vi "CSTK_Button_Icon_View.vi"(0 "Data In":T21 caption="数据输入", 2 "Display State In":T2={"ButtonSize"={"False"={"Width"=0, "Height"=0}, "True"={"Width"=0, "Height"=0}, "True to False"={"Width"=0, "Height"=0}, "False to True"={"Width"=0, "Height"=0}, "Hover in False"={"Width"=0, "Height"=0}, "Hover in True"={"Width"=0, "Height"=0}}, "Logo Image"={"False"={"image type"=0, "image depth"=0, "image"=[], "mask"=[], "colors"=[], "Rectangle"={"left"=0, "top"=0, "right"=0, "bottom"=0}}, "True"={"image type"=0, "image depth"=0, "image"=[], "mask"=[], "colors"=[], "Rectangle"={"left"=0, "top"=0, "right"=0, "bottom"=0}}, "True to False"={"image type"=0, "image depth"=0, "image"=[], "mask"=[], "colors"=[], "Rectangle"={"left"=0, "top"=0, "right"=0, "bottom"=0}}, "False to True"={"image type"=0, "image depth"=0, "image"=[], "mask"=[], "colors"=[], "Rectangle"={"left"=0, "top"=0, "right"=0, "bottom"=0}}, "Hover in False"={"image type"=0, "image depth"=0, "image"=[], "mask"=[], "colors"=[], "Rectangle"={"left"=0, "top"=0, "right"=0, "bottom"=0}}, "Hover in True"={"image type"=0, "image depth"=0, "image"=[], "mask"=[], "colors"=[], "Rectangle"={"left"=0, "top"=0, "right"=0, "bottom"=0}}}, "Logo Properties"={"False"={"Display Logo?"=FALSE, "Horizontal Offset"=0}, "True"={"Display Logo?"=FALSE, "Horizontal Offset"=0}, "True to False"={"Display Logo?"=FALSE, "Horizontal Offset"=0}, "False to True"={"Display Logo?"=FALSE, "Horizontal Offset"=0}, "Hover in False"={"Display Logo?"=FALSE, "Horizontal Offset"=0}, "Hover in True"={"Display Logo?"=FALSE, "Horizontal Offset"=0}}, "Text String"={"False"="", "True"="", "True to False"="", "False to True"="", "Hover in False"="", "Hover in True"=""}, "Text Properties"={"False"={"Display Text?"=FALSE, "Text Color"=0, "Horizontal Offset"=0, "Font Style"={"Font Name"="", "Size"=0, "Strikeout?"=FALSE, "Italic?"=FALSE, "Underline?"=FALSE, "Outline?"=FALSE, "Shadow?"=FALSE, "Bold?"=FALSE}}, "True"={"Display Text?"=FALSE, "Text Color"=0, "Horizontal Offset"=0, "Font Style"={"Font Name"="", "Size"=0, "Strikeout?"=FALSE, "Italic?"=FALSE, "Underline?"=FALSE, "Outline?"=FALSE, "Shadow?"=FALSE, "Bold?"=FALSE}}, "True to False"={"Display Text?"=FALSE, "Text Color"=0, "Horizontal Offset"=0, "Font Style"={"Font Name"="", "Size"=0, "Strikeout?"=FALSE, "Italic?"=FALSE, "Underline?"=FALSE, "Outline?"=FALSE, "Shadow?"=FALSE, "Bold?"=FALSE}}, "False to True"={"Display Text?"=FALSE, "Text Color"=0, "Horizontal Offset"=0, "Font Style"={"Font Name"="", "Size"=0, "Strikeout?"=FALSE, "Italic?"=FALSE, "Underline?"=FALSE, "Outline?"=FALSE, "Shadow?"=FALSE, "Bold?"=FALSE}}, "Hover in False"={"Display Text?"=FALSE, "Text Color"=0, "Horizontal Offset"=0, "Font Style"={"Font Name"="", "Size"=0, "Strikeout?"=FALSE, "Italic?"=FALSE, "Underline?"=FALSE, "Outline?"=FALSE, "Shadow?"=FALSE, "Bold?"=FALSE}}, "Hover in True"={"Display Text?"=FALSE, "Text Color"=0, "Horizontal Offset"=0, "Font Style"={"Font Name"="", "Size"=0, "Strikeout?"=FALSE, "Italic?"=FALSE, "Underline?"=FALSE, "Outline?"=FALSE, "Shadow?"=FALSE, "Bold?"=FALSE}}}, "BG Color"={"False"=0, "True"=0, "True to False"=0, "False to True"=0, "Hover in False"=0, "Hover in True"=0}, "Border Color"={"False"=0, "True"=0, "True to False"=0, "False to True"=0, "Hover in False"=0, "Hover in True"=0}, "Border Properties"={"False"={"Radius"=0, "Border Style"={"Width"=3, "Style"=enum."Solid"}}, "True"={"Radius"=0, "Border Style"={"Width"=3, "Style"=enum."Solid"}}, "True to False"={"Radius"=0, "Border Style"={"Width"=3, "Style"=enum."Solid"}}, "False to True"={"Radius"=0, "Border Style"={"Width"=3, "Style"=enum."Solid"}}, "Hover in False"={"Radius"=0, "Border Style"={"Width"=3, "Style"=enum."Solid"}}, "Hover in True"={"Radius"=0, "Border Style"={"Width"=3, "Style"=enum."Solid"}}}, "Current BG Image"={"False"=bytes[0], "True"=bytes[0], "True to False"=bytes[0], "False to True"=bytes[0], "Hover in False"=bytes[0], "Hover in True"=bytes[0]}, "DrawAreaSize"={"False"={"Width"=0, "Height"=0}, "True"={"Width"=0, "Height"=0}, "True to False"={"Width"=0, "Height"=0}, "False to True"={"Width"=0, "Height"=0}, "Hover in False"={"Width"=0, "Height"=0}, "Hover in True"={"Width"=0, "Height"=0}}, "Text String Offset"={"False"=0, "True"=0, "True to False"=0, "False to True"=0, "Hover in False"=0, "Hover in True"=0}} caption="显示状态输入", 3 "Container State":T20 caption="容器状态") -> (6 "Data Out":T21 caption="数据输出", 7 "Display State Out":T2={"ButtonSize"={"False"={"Width"=0, "Height"=0}, "True"={"Width"=0, "Height"=0}, "True to False"={"Width"=0, "Height"=0}, "False to True"={"Width"=0, "Height"=0}, "Hover in False"={"Width"=0, "Height"=0}, "Hover in True"={"Width"=0, "Height"=0}}, "Logo Image"={"False"={"image type"=0, "image depth"=0, "image"=[], "mask"=[], "colors"=[], "Rectangle"={"left"=0, "top"=0, "right"=0, "bottom"=0}}, "True"={"image type"=0, "image depth"=0, "image"=[], "mask"=[], "colors"=[], "Rectangle"={"left"=0, "top"=0, "right"=0, "bottom"=0}}, "True to False"={"image type"=0, "image depth"=0, "image"=[], "mask"=[], "colors"=[], "Rectangle"={"left"=0, "top"=0, "right"=0, "bottom"=0}}, "False to True"={"image type"=0, "image depth"=0, "image"=[], "mask"=[], "colors"=[], "Rectangle"={"left"=0, "top"=0, "right"=0, "bottom"=0}}, "Hover in False"={"image type"=0, "image depth"=0, "image"=[], "mask"=[], "colors"=[], "Rectangle"={"left"=0, "top"=0, "right"=0, "bottom"=0}}, "Hover in True"={"image type"=0, "image depth"=0, "image"=[], "mask"=[], "colors"=[], "Rectangle"={"left"=0, "top"=0, "right"=0, "bottom"=0}}}, "Logo Properties"={"False"={"Display Logo?"=FALSE, "Horizontal Offset"=0}, "True"={"Display Logo?"=FALSE, "Horizontal Offset"=0}, "True to False"={"Display Logo?"=FALSE, "Horizontal Offset"=0}, "False to True"={"Display Logo?"=FALSE, "Horizontal Offset"=0}, "Hover in False"={"Display Logo?"=FALSE, "Horizontal Offset"=0}, "Hover in True"={"Display Logo?"=FALSE, "Horizontal Offset"=0}}, "Text String"={"False"="", "True"="", "True to False"="", "False to True"="", "Hover in False"="", "Hover in True"=""}, "Text Properties"={"False"={"Display Text?"=FALSE, "Text Color"=0, "Horizontal Offset"=0, "Font Style"={"Font Name"="", "Size"=0, "Strikeout?"=FALSE, "Italic?"=FALSE, "Underline?"=FALSE, "Outline?"=FALSE, "Shadow?"=FALSE, "Bold?"=FALSE}}, "True"={"Display Text?"=FALSE, "Text Color"=0, "Horizontal Offset"=0, "Font Style"={"Font Name"="", "Size"=0, "Strikeout?"=FALSE, "Italic?"=FALSE, "Underline?"=FALSE, "Outline?"=FALSE, "Shadow?"=FALSE, "Bold?"=FALSE}}, "True to False"={"Display Text?"=FALSE, "Text Color"=0, "Horizontal Offset"=0, "Font Style"={"Font Name"="", "Size"=0, "Strikeout?"=FALSE, "Italic?"=FALSE, "Underline?"=FALSE, "Outline?"=FALSE, "Shadow?"=FALSE, "Bold?"=FALSE}}, "False to True"={"Display Text?"=FALSE, "Text Color"=0, "Horizontal Offset"=0, "Font Style"={"Font Name"="", "Size"=0, "Strikeout?"=FALSE, "Italic?"=FALSE, "Underline?"=FALSE, "Outline?"=FALSE, "Shadow?"=FALSE, "Bold?"=FALSE}}, "Hover in False"={"Display Text?"=FALSE, "Text Color"=0, "Horizontal Offset"=0, "Font Style"={"Font Name"="", "Size"=0, "Strikeout?"=FALSE, "Italic?"=FALSE, "Underline?"=FALSE, "Outline?"=FALSE, "Shadow?"=FALSE, "Bold?"=FALSE}}, "Hover in True"={"Display Text?"=FALSE, "Text Color"=0, "Horizontal Offset"=0, "Font Style"={"Font Name"="", "Size"=0, "Strikeout?"=FALSE, "Italic?"=FALSE, "Underline?"=FALSE, "Outline?"=FALSE, "Shadow?"=FALSE, "Bold?"=FALSE}}}, "BG Color"={"False"=0, "True"=0, "True to False"=0, "False to True"=0, "Hover in False"=0, "Hover in True"=0}, "Border Color"={"False"=0, "True"=0, "True to False"=0, "False to True"=0, "Hover in False"=0, "Hover in True"=0}, "Border Properties"={"False"={"Radius"=0, "Border Style"={"Width"=3, "Style"=enum."Solid"}}, "True"={"Radius"=0, "Border Style"={"Width"=3, "Style"=enum."Solid"}}, "True to False"={"Radius"=0, "Border Style"={"Width"=3, "Style"=enum."Solid"}}, "False to True"={"Radius"=0, "Border Style"={"Width"=3, "Style"=enum."Solid"}}, "Hover in False"={"Radius"=0, "Border Style"={"Width"=3, "Style"=enum."Solid"}}, "Hover in True"={"Radius"=0, "Border Style"={"Width"=3, "Style"=enum."Solid"}}}, "Current BG Image"={"False"=bytes[0], "True"=bytes[0], "True to False"=bytes[0], "False to True"=bytes[0], "Hover in False"=bytes[0], "Hover in True"=bytes[0]}, "DrawAreaSize"={"False"={"Width"=0, "Height"=0}, "True"={"Width"=0, "Height"=0}, "True to False"={"Width"=0, "Height"=0}, "False to True"={"Width"=0, "Height"=0}, "Hover in False"={"Width"=0, "Height"=0}, "Hover in True"={"Width"=0, "Height"=0}}, "Text String Offset"={"False"=0, "True"=0, "True to False"=0, "False to True"=0, "Hover in False"=0, "Hover in True"=0}} caption="显示状态输出", 8 "Action":T1 caption="动作")   [LabVIEW 2015, in "CSTK_Button_Icon.xctl"]
uses:
  CSTK_Button_Icon.xctl
  CSTK_Button_Icon_Data.ctl
  <vilib>/_xctls/Container State.ctl
  CSTK_Button_Icon_Status.ctl
  Private/TypeDefinitions/_CSTK_Button_Icon_ButtonSize.ctl
  <vilib>/Utility/miscctls.llb/LVBoundsTypeDef.ctl
  Private/TypeDefinitions/_CSTK_Button_Icon_LogoImage.ctl
  <vilib>/picture/picture.llb/imagedata.ctl
  Private/TypeDefinitions/_CSTK_Button_Icon_LogoProperties.ctl
  Private/TypeDefinitions/_CSTK_Button_Icon_LogoProperties_Data.ctl
  Private/TypeDefinitions/_CSTK_Button_Icon_TextString.ctl
  Private/TypeDefinitions/_CSTK_Button_Icon_TextProperties.ctl
  Private/TypeDefinitions/_CSTK_Button_Icon_TextProperties_Data.ctl
  Private/TypeDefinitions/_CSTK_Button_Icon_TextProperties_FontStyle.ctl
  Private/TypeDefinitions/_CSTK_Button_Icon_BGColor.ctl
  Private/TypeDefinitions/_CSTK_Button_Icon_BorderColor.ctl
  Private/TypeDefinitions/_CSTK_Button_Icon_BorderProperties.ctl
  Private/TypeDefinitions/_CSTK_Button_Icon_BorderProperties_Data.ctl
  Private/TypeDefinitions/_CSTK_Button_Icon_CurrentBGImage.ctl
  Private/TypeDefinitions/_CSTK_Button_Icon_DrawAreaSize.ctl
  Private/TypeDefinitions/_CSTK_Button_Icon_TextStartOffset.ctl
  <vilib>/_xctls/Action.ctl
  Private/TypeDefinitions/_CSTK_Button_Icon_EventData.ctl
  <vilib>/_xctls/XControlSupport.lvlib
panel:
  out "CSTK_Button":picture
types:
  T1 = typedef "XControlSupport.lvlib/Action.ctl" = cluster{"Data Changed?":bool, "State Changed?":bool, "Action Name":string}
  T2 = typedef "CSTK_Button_Icon.xctl/CSTK_Button_Icon_Status.ctl" = cluster{"ButtonSize":T3, "Logo Image":T5, "Logo Properties":T7, "Text String":T9, "Text Properties":T10, "BG Color":T13, "Border Color":T14, "Border Properties":T15, "Current BG Image":T17, "DrawAreaSize":T18, "Text String Offset":T19}
  T3 = typedef "CSTK_Button_Icon.xctl/_CSTK_Button_Icon_ButtonSize.ctl" = cluster{"False":T4, "True":T4, "True to False":T4, "False to True":T4, "Hover in False":T4, "Hover in True":T4}
  T4 = typedef "LVBoundsTypeDef.ctl" = cluster{"Width":u32, "Height":u32}
  T5 = typedef "CSTK_Button_Icon.xctl/_CSTK_Button_Icon_LogoImage.ctl" = cluster{"False":T6, "True":T6, "True to False":T6, "False to True":T6, "Hover in False":T6, "Hover in True":T6}
  T6 = typedef "imagedata.ctl" = cluster{"image type":i32, "image depth":i32, "image":u8[], "mask":u8[], "colors":u32[], "Rectangle":cluster{"left":i16, "top":i16, "right":i16, "bottom":i16}}
  T7 = typedef "CSTK_Button_Icon.xctl/_CSTK_Button_Icon_LogoProperties.ctl" = cluster{"False":T8, "True":T8, "True to False":T8, "False to True":T8, "Hover in False":T8, "Hover in True":T8}
  T8 = typedef "CSTK_Button_Icon.xctl/_CSTK_Button_Icon_LogoProperties_Data.ctl" = cluster{"Display Logo?":bool, "Horizontal Offset":i16}
  T9 = typedef "CSTK_Button_Icon.xctl/_CSTK_Button_Icon_TextString.ctl" = cluster{"False":string, "True":string, "True to False":string, "False to True":string, "Hover in False":string, "Hover in True":string}
  T10 = typedef "CSTK_Button_Icon.xctl/_CSTK_Button_Icon_TextProperties.ctl" = cluster{"False":T11, "True":T11, "True to False":T11, "False to True":T11, "Hover in False":T11, "Hover in True":T11}
  T11 = typedef "CSTK_Button_Icon.xctl/_CSTK_Button_Icon_TextProperties_Data.ctl" = cluster{"Display Text?":bool, "Text Color":u32, "Horizontal Offset":i16, "Font Style":T12}
  T12 = typedef "CSTK_Button_Icon.xctl/_CSTK_Button_Icon_TextProperties_FontStyle.ctl" = cluster{"Font Name":string, "Size":i16, "Strikeout?":bool, "Italic?":bool, "Underline?":bool, "Outline?":bool, "Shadow?":bool, "Bold?":bool}
  T13 = typedef "CSTK_Button_Icon.xctl/_CSTK_Button_Icon_BGColor.ctl" = cluster{"False":u32, "True":u32, "True to False":u32, "False to True":u32, "Hover in False":u32, "Hover in True":u32}
  T14 = typedef "CSTK_Button_Icon.xctl/_CSTK_Button_Icon_BorderColor.ctl" = cluster{"False":u32, "True":u32, "True to False":u32, "False to True":u32, "Hover in False":u32, "Hover in True":u32}
  T15 = typedef "CSTK_Button_Icon.xctl/_CSTK_Button_Icon_BorderProperties.ctl" = cluster{"False":T16, "True":T16, "True to False":T16, "False to True":T16, "Hover in False":T16, "Hover in True":T16}
  T16 = typedef "CSTK_Button_Icon.xctl/_CSTK_Button_Icon_BorderProperties_Data.ctl" = cluster{"Radius":i16, "Border Style":cluster{"Width":u16, "Style":enum32{"Solid", "Dash", "Dot", "DashDot", "DashDotDot"}}}
  T17 = typedef "CSTK_Button_Icon.xctl/_CSTK_Button_Icon_CurrentBGImage.ctl" = cluster{"False":picture, "True":picture, "True to False":picture, "False to True":picture, "Hover in False":picture, "Hover in True":picture}
  T18 = typedef "CSTK_Button_Icon.xctl/_CSTK_Button_Icon_DrawAreaSize.ctl" = cluster{"False":T4, "True":T4, "True to False":T4, "False to True":T4, "Hover in False":T4, "Hover in True":T4}
  T19 = typedef "CSTK_Button_Icon.xctl/_CSTK_Button_Icon_TextStartOffset.ctl" = cluster{"False":i32, "True":i32, "True to False":i32, "False to True":i32, "Hover in False":i32, "Hover in True":i32}
  T20 = typedef "XControlSupport.lvlib/Container State.ctl" = cluster{"Indicator?":bool, "Run Mode?":bool, " Refnum":refnum<vi>}
  T21 = typedef "CSTK_Button_Icon.xctl/CSTK_Button_Icon_Data.ctl" = bool
  T22 = typedef "CSTK_Button_Icon.xctl/_CSTK_Button_Icon_EventData.ctl" = cluster{"BGImage":picture, "DrawAreaSize":T4, "UpdateDrawArea":bool, "调用方":string}
  T23 = typedef "LVRectTypeDef.ctl" = cluster{"Left":i16, "Top":i16, "Right":i16, "Bottom":i16}
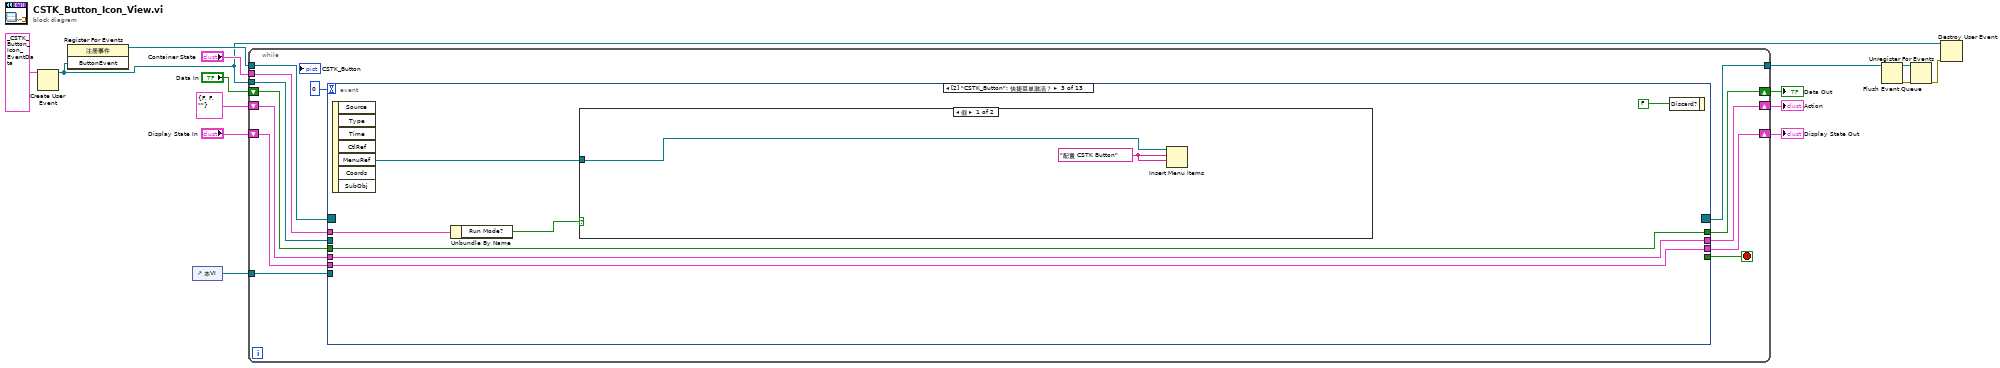
[diagram p0: block diagram]
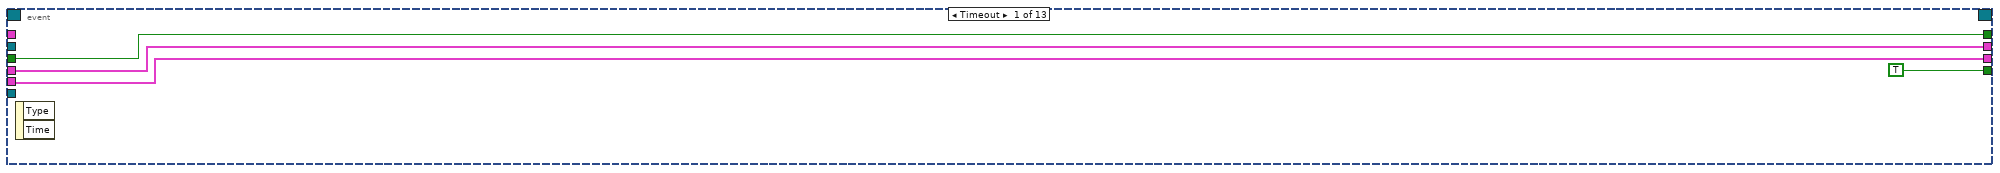
[diagram p2: hidden frame]
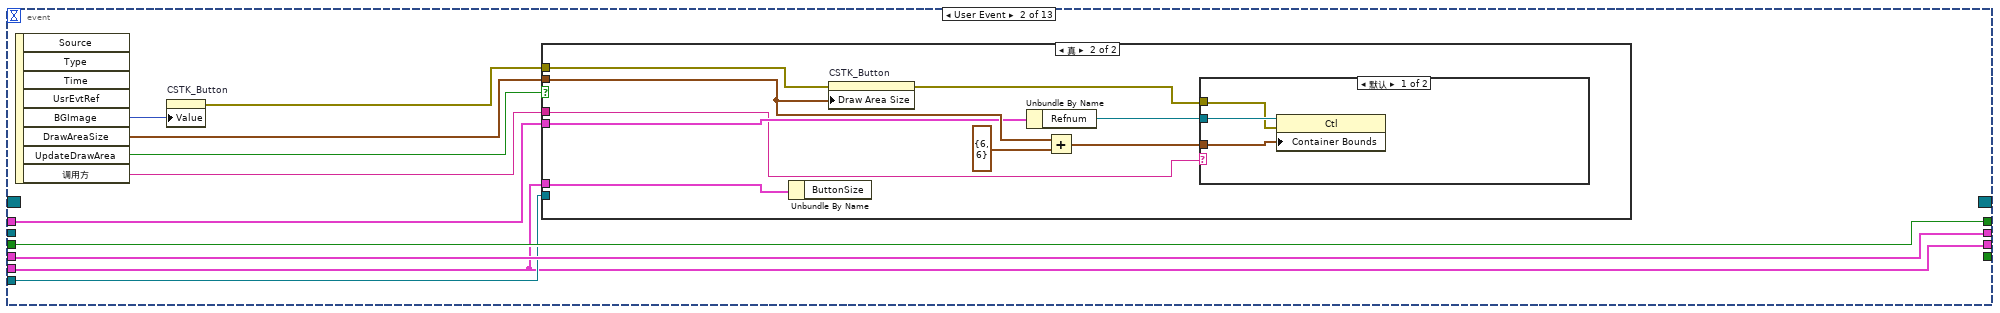
[diagram p3: hidden frame]
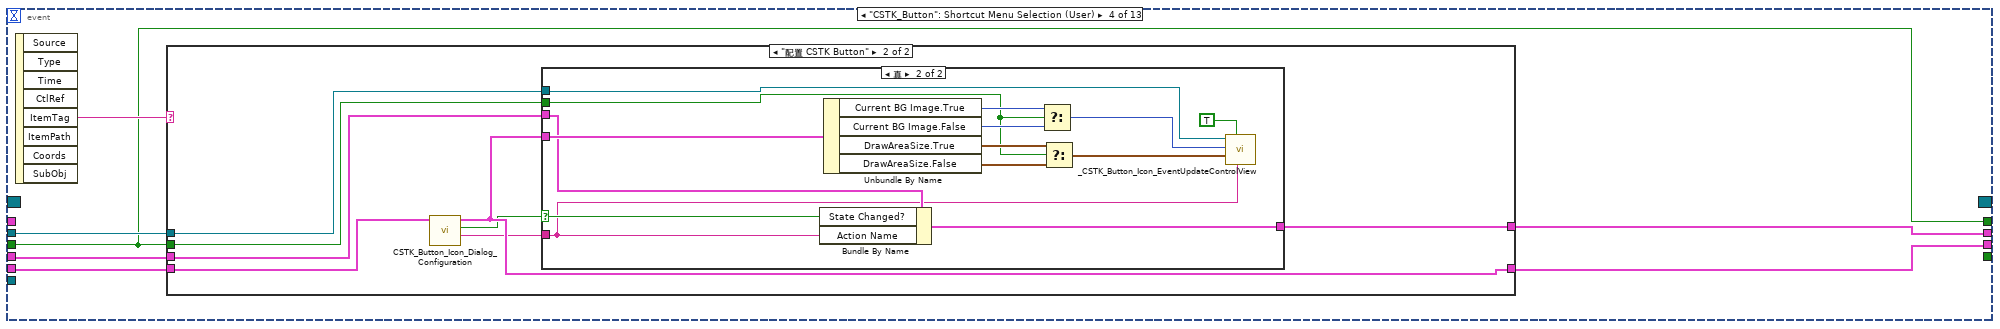
[diagram p7: hidden frame]
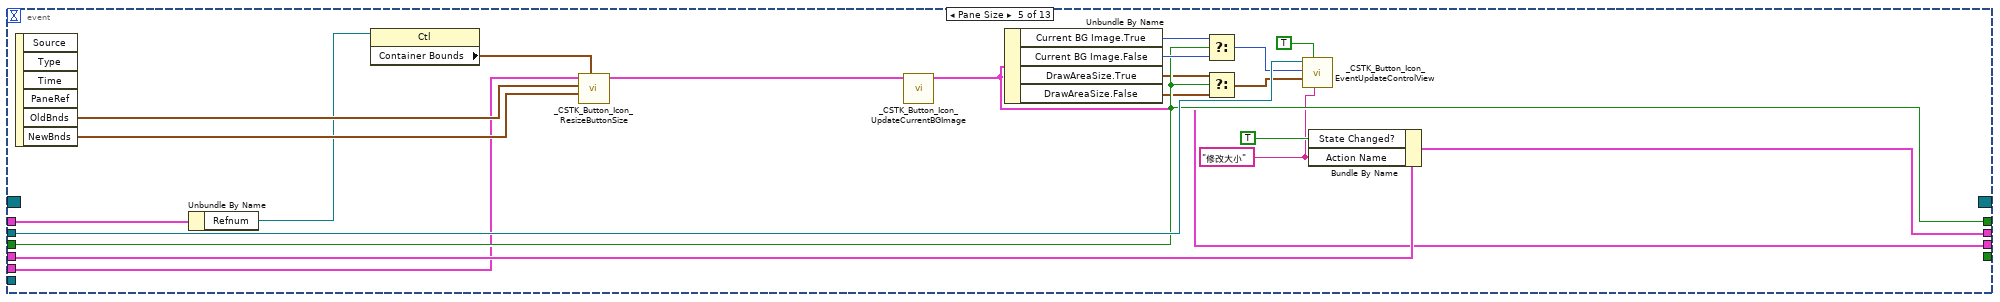
[diagram p10: hidden frame]
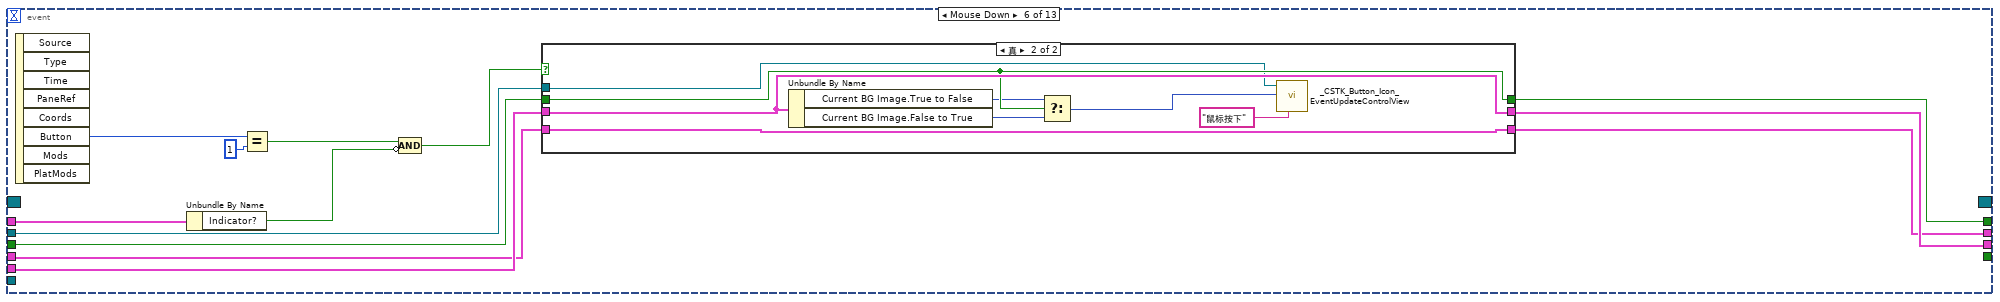
[diagram p11: hidden frame]
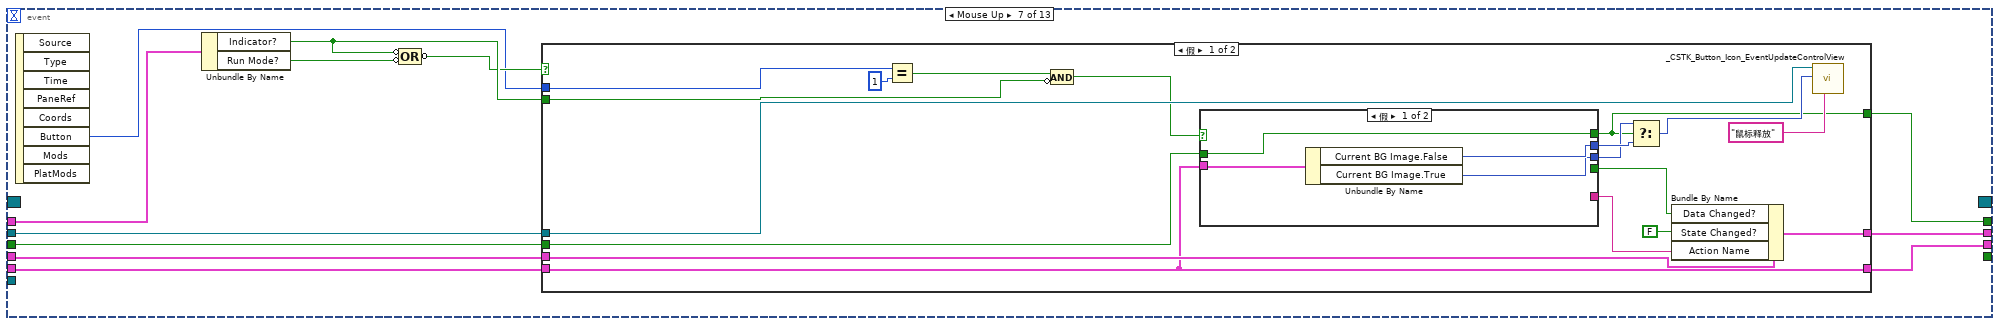
[diagram p13: hidden frame]
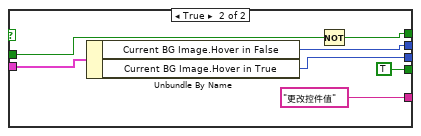
[diagram p14: hidden frame]
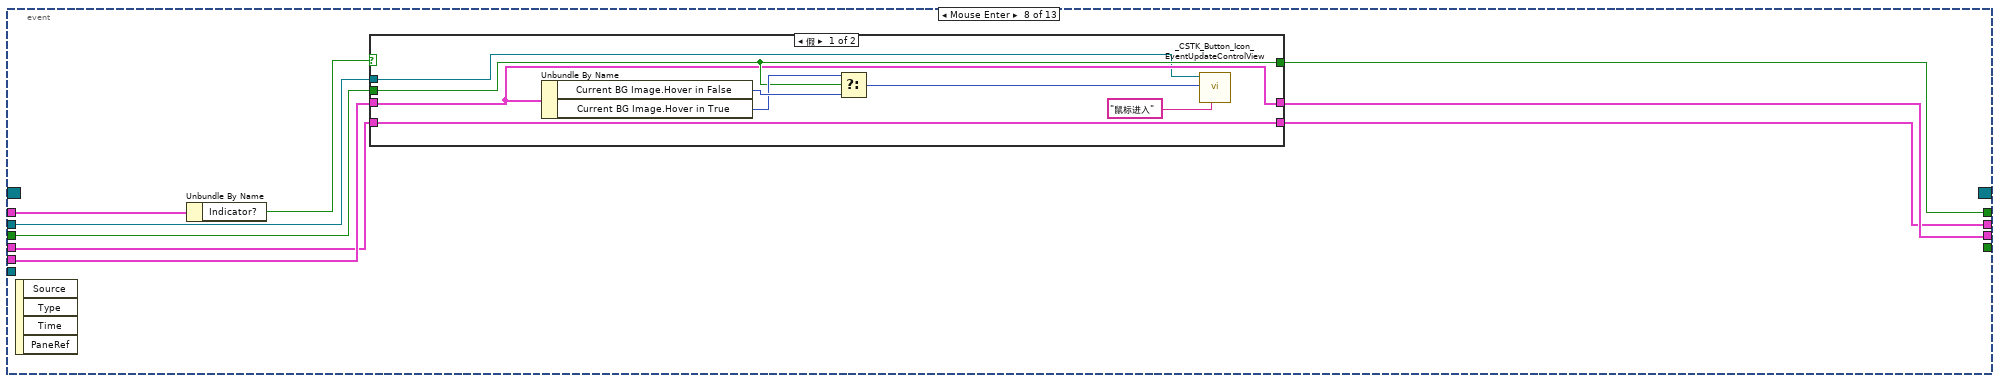
[diagram p16: hidden frame]
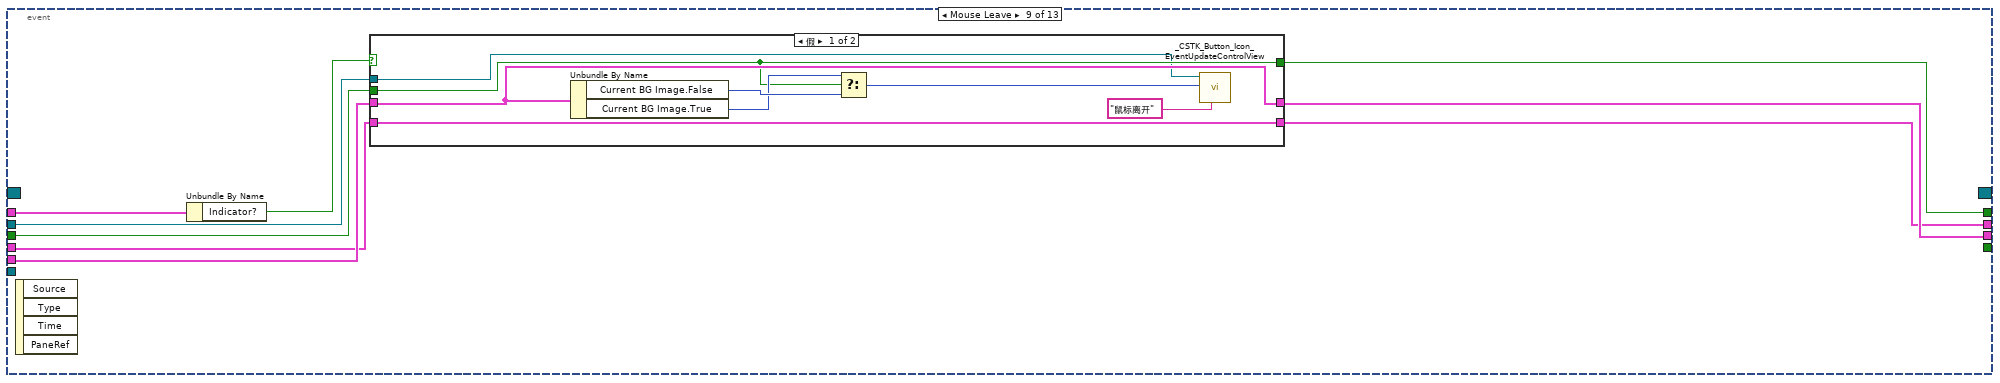
[diagram p18: hidden frame]
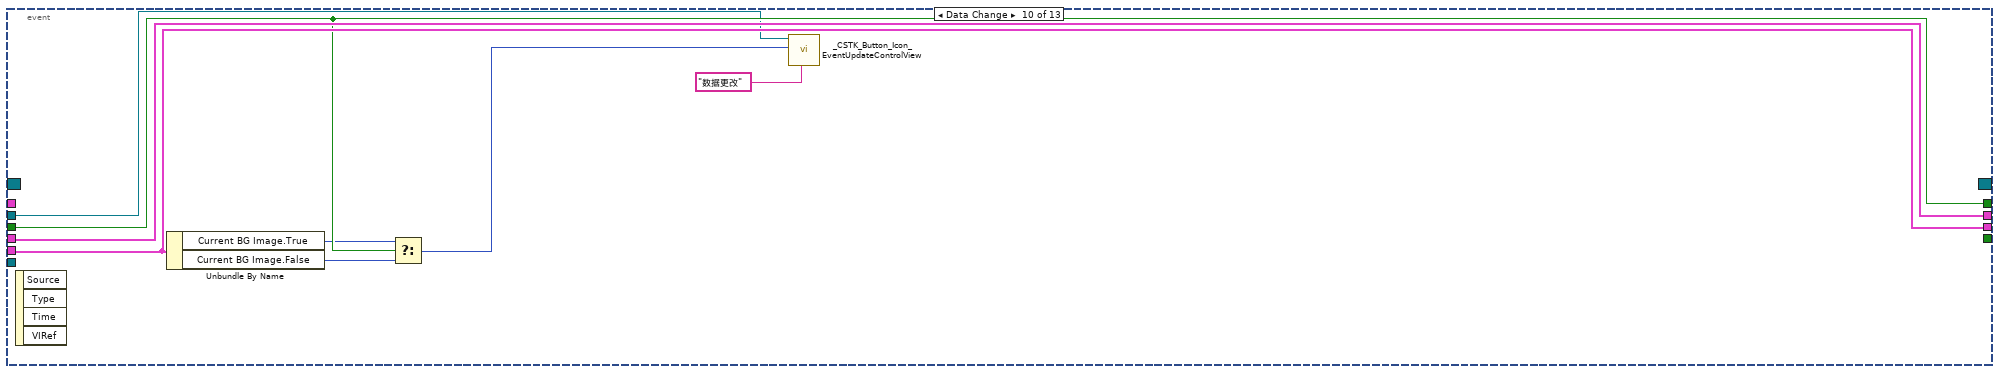
[diagram p20: hidden frame]
diagram:
  n1 = Create User Event(user event datatype=T22 {"BGImage"=bytes[0], "DrawAreaSize"={"Width"=0, "Height"=0}, "UpdateDrawArea"=FALSE, "调用方"=""} ("ButtonEvent")) -> (user event=w2:refnum<user-event>)  [unwired: 1 in, 1 out]
  n2 = register-events(w2) -> (reference out=w6:refnum<event-registration>)  [unwired: 2 in, 1 out]
  n3 = control-ref of="本VI"() -> (w8:refnum<vi>)
  n4 = while {
    shift-right: [w27] -> w12
    shift-left: "Display State In" -> [w28]
    tunnel: "Container State" -> [w24]
    shift-right: [w22] -> w15
    shift-left: "Data In" -> [w23]
    shift-right: [w20] -> w10
    shift-left: T1 {"Data Changed?"=FALSE, "State Changed?"=FALSE, "Action Name"=""} ("Action") -> [w21]
    tunnel: w8 -> [w19]
    tunnel: w6 -> [w18]
    tunnel: w2 -> [w16]
    tunnel: [w17] -> w5
    stop <- w26 stop-if-true
    n5 = event shown="[2] \"CSTK_Button\": 快捷菜单激活？" {
      selector: w18 -> [_ _ _ _ _ _ _ _ _ _ _ _ _]
      dyn-events: [_ _ _ _ _ _ _ _ _ _ _ _ _] -> w17
      timeout: 0 -> [_ _ _ _ _ _ _ _ _ _ _ _ _]
      tunnel: w28 -> [w30 w33 w61 w69 w102 w127 w150 w191 w211 w231 w233 w245 w257]
      tunnel: [w30 w33 w61 w68 w100 w126 w149 w190 w210 w231 w233 w245 w257] -> w27
      tunnel: [TRUE _ _ _ _ _ _ _ _ _ _ _ _] -> w26
      tunnel: w24 -> [_ w35 w56 _ w99 w123 w146 w187 w207 _ _ w251 w258]
      tunnel: w23 -> [w29 w42 w60 w66 w107 w129 w152 w193 w213 w230 w243 w250 w256]
      tunnel: [w29 w42 w60 w66 w107 w128 w151 w192 w212 w230 w243 w250 w256] -> w22
      tunnel: [w31 w41 w59 w64 w115 w124 w147 w188 w208 w232 w244 w248 w254] -> w20
      tunnel: w21 -> [w31 w41 w59 w65 w116 w125 w148 w189 w209 w232 w244 w249 w255]
      tunnel: w19 -> [_ w36 _ _ _ _ _ _ _ _ _ _ _]
      tunnel: w16 -> [_ _ _ w67 w111 w121 w142 w185 w205 w227 w238 _ _]
      event Timeout {
        n6 = event-data() -> ()  [unwired: 1 in, 2 out]
      }
      event User Event {
        n7 = event-data() -> ("BGImage"=w40:picture, "DrawAreaSize"=w38:T4, "UpdateDrawArea"=w37:bool, "调用方"=w34:string)  [unwired: 1 in, 4 out]
        n8 = property on="CSTK_Button" class="Pict"("Value"=w40) -> (error out=w39:errorcluster)  [unwired: 2 in, 1 out]
        n9 = case shown="真" w37 {
          tunnel: w39 -> [_ w51]
          tunnel: w38 -> [_ w49]
          tunnel: w36 -> [_ _]
          tunnel: w35 -> [_ w48]
          tunnel: w34 -> [_ w44]
          tunnel: w33 -> [_ w43]
          frame False {
          }
          frame True {
            n10 = Unbundle By Name(w43) -> ()  [unwired: 1 out]
            n11 = property on="CSTK_Button" class="Pict"(error in=w51, "Draw Area Size"=w49) -> (error out=w46:errorcluster)  [unwired: 1 in, 1 out]
            n12 = Unbundle By Name(w48) -> ("Refnum"=w45:refnum<vi>)
            n13 = Add(x=w49, y=T4 {"Width"=6, "Height"=6}) -> (x+y=w47:T4)
            n14 = case shown="默认" w44 {
              tunnel: w47 -> [w52 _]
              tunnel: w45 -> [w54 _]
              tunnel: w46 -> [w53 _]
              frame Default {
                n15 = property class="Ctl"(reference=w54, error in=w53, "Container Bounds"=w52) -> ()  [unwired: 2 out]
              }
              frame "修改大小" {
              }
            }
          }
        }
      }
      event "CSTK_Button": Shortcut Menu Activation? {
        n16 = event-data() -> ("MenuRef"=w58:refnum<k9>)  [unwired: 1 in, 6 out]
        n17 = Unbundle By Name(w56) -> ("Run Mode?"=w55:bool)
        n18 = case shown="假" w55 {
          tunnel: w58 -> [w62 _]
          frame False {
            w63 = "配置 CSTK Button"
            n19 = Insert Menu Items(7:w63, 8:w63, 9:w62) -> ()  [unwired: 3 in, 3 out]
          }
          frame True {
          }
        }
        n20 = event-data("Discard?"=FALSE ("放弃？")) -> ()  [unwired: 1 in, 1 out]
      }
      event "CSTK_Button": Shortcut Menu Selection (User) {
        n21 = event-data() -> ("ItemTag"=w70:string)  [unwired: 1 in, 7 out]
        n22 = case shown="\"配置 CSTK Button\"" w70 {
          tunnel: w69 -> [w72 w80]
          tunnel: [w72 w78] -> w68
          tunnel: w67 -> [_ w79]
          tunnel: w66 -> [_ w77]
          tunnel: [w71 w73] -> w64
          tunnel: w65 -> [w71 w74]
          frame Default {
          }
          frame "配置 CSTK Button" {
            n23 = call "CSTK_Button_Icon_Dialog_Configuration.vi"("State in"=w80) -> ("Action Name"=w76:string, "State Changed?"=w75:bool, "State out"=w78:T2)  [unwired: 8 in]
            n24 = case shown="真" w75 {
              selector: w75 -> [_ w84]
              tunnel: w79 -> [_ w88]
              tunnel: w78 -> [_ w87]
              tunnel: w76 -> [_ w83]
              tunnel: w77 -> [_ w86]
              tunnel: w74 -> [w81 w85]
              tunnel: [w81 w82] -> w73
              frame False {
              }
              frame True {
                n25 = Bundle By Name(cluster=w85, "State Changed?"=w84, "Action Name"=w83) -> (w82:T1)
                n26 = Unbundle By Name(w87) -> ("Current BG Image.True"=w95:picture, "Current BG Image.False"=w94:picture, "DrawAreaSize.True"=w93:T4, "DrawAreaSize.False"=w92:T4)
                n27 = Select(t=w95, s=w86, f=w94) -> (s? t:f=w91:picture)
                n28 = Select(t=w93, s=w86, f=w92) -> (s? t:f=w90:T4)
                n29 = call "_CSTK_Button_Icon_EventUpdateControlView.vi"("调用方"=w83, "UpdateDrawArea"=TRUE, "DrawAreaSize"=w90, "BGImage"=w91, "用户事件输入"=w88) -> ()  [unwired: 5 in, 2 out]
              }
            }
          }
        }
      }
      event Pane Size {
        w96 = "修改大小" ("Action Name")
        n30 = event-data() -> ("OldBnds"=w113:T23, "NewBnds"=w112:T23)  [unwired: 1 in, 4 out]
        n31 = Unbundle By Name(w99) -> ("Refnum"=w98:refnum<vi>)
        n32 = property class="Ctl"(reference=w98) -> ("Container Bounds"=w97:T4)  [unwired: 1 in, 2 out]
        n33 = call "_CSTK_Button_Icon_ResizeButtonSize.vi"("XControl:容器边界"=w97, "NewBnds"=w112, "OldBnds"=w113, "Display State 输入"=w102) -> ("Display State 输出"=w101:T2)  [unwired: 7 in]
        n34 = call "_CSTK_Button_Icon_UpdateCurrentBGImage.vi"("State in"=w101) -> ("State out"=w100:T2)  [unwired: 10 in]
        n35 = Unbundle By Name(w100) -> ("Current BG Image.True"=w110:picture, "Current BG Image.False"=w109:picture, "DrawAreaSize.True"=w106:T4, "DrawAreaSize.False"=w105:T4)
        n36 = Select(t=w110, s=w107, f=w109) -> (s? t:f=w108:picture)
        n37 = Select(t=w106, s=w107, f=w105) -> (s? t:f=w104:T4)
        n38 = call "_CSTK_Button_Icon_EventUpdateControlView.vi"("调用方"=w96, "UpdateDrawArea"=TRUE, "DrawAreaSize"=w104, "BGImage"=w108, "用户事件输入"=w111) -> ()  [unwired: 5 in, 2 out]
        n39 = Bundle By Name(cluster=w116, "State Changed?"=TRUE, "Action Name"=w96) -> (w115:T1)
      }
      event Mouse Down {
        n40 = event-data() -> ("Button"=w119:u16)  [unwired: 1 in, 7 out]
        n41 = Unbundle By Name(w123) -> ("Indicator?"=w122:bool)
        n42 = Equal?(x=w119, y=u16 1) -> (x = y?=w117:bool)
        n43 = Compound Arithmetic op=AND ("复合运算")(w117, invert w122) -> (w120:bool)
        n44 = case shown="真" w120 {
          tunnel: w129 -> [w132 w139]
          tunnel: [w132 w139] -> w128
          tunnel: w127 -> [w131 w140]
          tunnel: [w131 w140] -> w126
          tunnel: w125 -> [w130 w136]
          tunnel: [w130 w136] -> w124
          tunnel: w121 -> [_ w135]
          frame False {
          }
          frame True {
            n45 = Unbundle By Name(w140) -> ("Current BG Image.True to False"=w138:picture, "Current BG Image.False to True"=w137:picture)
            n46 = Select(t=w138, s=w139, f=w137) -> (s? t:f=w134:picture)
            n47 = call "_CSTK_Button_Icon_EventUpdateControlView.vi"("调用方"="鼠标按下", "BGImage"=w134, "用户事件输入"=w135) -> ()  [unwired: 7 in, 2 out]
          }
        }
      }
      event Mouse Up {
        n48 = event-data() -> ("Button"=w141:u16)  [unwired: 1 in, 7 out]
        n49 = Unbundle By Name(w146) -> ("Indicator?"=w145:bool, "Run Mode?"=w144:bool)
        n50 = Compound Arithmetic op=OR ("复合运算")(invert w145, invert w144) -> (invert w143:bool)
        n51 = case shown="假" w143 {
          tunnel: w152 -> [w156 w184]
          tunnel: [w155 w184] -> w151
          tunnel: w150 -> [w167 w183]
          tunnel: [w167 w183] -> w149
          tunnel: w148 -> [w170 w182]
          tunnel: [w169 w182] -> w147
          tunnel: w145 -> [w164 _]
          tunnel: w142 -> [w163 _]
          tunnel: w141 -> [w159 _]
          frame False {
            n52 = Equal?(x=w159, y=u16 1) -> (x = y?=w157:bool)
            n53 = Compound Arithmetic op=AND ("复合运算")(w157, invert w164) -> (w160:bool)
            n54 = case shown="假" w160 {
              tunnel: w167 -> [w174 w181]
              tunnel: [w173 w180] -> w166
              tunnel: [w172 w179] -> w165
              tunnel: w156 -> [w171 w178]
              tunnel: [w171 w177] -> w155
              tunnel: [_ TRUE ("Data Changed?")] -> w154
              tunnel: [_ "更改控件值" ("Action Name")] -> w153
              frame False {
                n55 = Unbundle By Name(w174) -> ("Current BG Image.False"=w173:picture, "Current BG Image.True"=w172:picture)
              }
              frame True {
                n56 = Unbundle By Name(w181) -> ("Current BG Image.Hover in False"=w180:picture, "Current BG Image.Hover in True"=w179:picture)
                n57 = Not(x=w178) -> (.not. x?=w177:T21)
              }
            }
            n58 = Select(t=w165, s=w155, f=w166) -> (s? t:f=w162:picture)
            n59 = Bundle By Name(cluster=w170, "Data Changed?"=w154, "State Changed?"=FALSE, "Action Name"=w153) -> (w169:T1)
            n60 = call "_CSTK_Button_Icon_EventUpdateControlView.vi"("调用方"="鼠标释放", "BGImage"=w162, "用户事件输入"=w163) -> ()  [unwired: 7 in, 2 out]
          }
          frame True {
          }
        }
      }
      event Mouse Enter {
        n61 = event-data() -> ()  [unwired: 1 in, 4 out]
        n62 = Unbundle By Name(w187) -> ("Indicator?"=w186:bool)
        n63 = case shown="假" w186 {
          tunnel: w193 -> [w198 w204]
          tunnel: [w198 w204] -> w192
          tunnel: w191 -> [w197 w203]
          tunnel: [w197 w203] -> w190
          tunnel: w189 -> [w201 w202]
          tunnel: [w201 w202] -> w188
          tunnel: w185 -> [w195 _]
          frame False {
            n64 = Unbundle By Name(w197) -> ("Current BG Image.Hover in False"=w200:picture, "Current BG Image.Hover in True"=w199:picture)
            n65 = Select(t=w199, s=w198, f=w200) -> (s? t:f=w196:picture)
            n66 = call "_CSTK_Button_Icon_EventUpdateControlView.vi"("调用方"="鼠标进入", "BGImage"=w196, "用户事件输入"=w195) -> ()  [unwired: 7 in, 2 out]
          }
          frame True {
          }
        }
      }
      event Mouse Leave {
        n67 = event-data() -> ()  [unwired: 1 in, 4 out]
        n68 = Unbundle By Name(w207) -> ("Indicator?"=w206:bool)
        n69 = case shown="假" w206 {
          tunnel: w213 -> [w217 w224]
          tunnel: [w217 w224] -> w212
          tunnel: w211 -> [w220 w223]
          tunnel: [w220 w223] -> w210
          tunnel: w209 -> [w221 w222]
          tunnel: [w221 w222] -> w208
          tunnel: w205 -> [w215 _]
          frame False {
            n70 = Unbundle By Name(w220) -> ("Current BG Image.False"=w219:picture, "Current BG Image.True"=w218:picture)
            n71 = Select(t=w218, s=w217, f=w219) -> (s? t:f=w216:picture)
            n72 = call "_CSTK_Button_Icon_EventUpdateControlView.vi"("调用方"="鼠标离开", "BGImage"=w216, "用户事件输入"=w215) -> ()  [unwired: 7 in, 2 out]
          }
          frame True {
          }
        }
      }
      event Data Change {
        n73 = event-data() -> ()  [unwired: 1 in, 4 out]
        n74 = Unbundle By Name(w231) -> ("Current BG Image.True"=w229:picture, "Current BG Image.False"=w228:picture)
        n75 = Select(t=w229, s=w230, f=w228) -> (s? t:f=w226:picture)
        n76 = call "_CSTK_Button_Icon_EventUpdateControlView.vi"("调用方"="数据更改", "BGImage"=w226, "用户事件输入"=w227) -> ()  [unwired: 7 in, 2 out]
      }
      event Display State Change {
        n77 = event-data() -> ()  [unwired: 1 in, 4 out]
        n78 = Unbundle By Name(w233) -> ("Current BG Image.True"=w242:picture, "Current BG Image.False"=w241:picture, "DrawAreaSize.True"=w240:T4, "DrawAreaSize.False"=w239:T4)
        n79 = Select(t=w242, s=w243, f=w241) -> (s? t:f=w237:picture)
        n80 = Select(t=w240, s=w243, f=w239) -> (s? t:f=w236:T4)
        n81 = call "_CSTK_Button_Icon_EventUpdateControlView.vi"("调用方"="显示状态更改", "UpdateDrawArea"=TRUE, "DrawAreaSize"=w236, "BGImage"=w237, "用户事件输入"=w238) -> ()  [unwired: 5 in, 2 out]
      }
      event Direction Change {
        n82 = event-data() -> ()  [unwired: 1 in, 4 out]
        n83 = Unbundle By Name(w251) -> ()  [unwired: 1 out]
        n84 = Bundle By Name(cluster=w249, "State Changed?"=TRUE, "Action Name"="修改方向") -> (w248:T1)
      }
      event Exec State Change {
        n85 = event-data() -> ()  [unwired: 1 in, 4 out]
        n86 = Unbundle By Name(w258) -> ()  [unwired: 1 out]
        n87 = Bundle By Name(cluster=w255, "State Changed?"=TRUE, "Action Name"="更新控件") -> (w254:T1)
      }
    }
  }
  "Display State Out" <- w12
  "Data Out" <- w15
  "Action" <- w10
  n88 = Flush Event Queue(0:w5) -> (8:w4:refnum<event-registration>, 11:w3:errorcluster)  [unwired: 5 in, 1 out]
  n89 = Unregister For Events(event registration refnum=w4, error in=w3) -> (error out=w1:errorcluster)
  n90 = Destroy User Event(user event=w2, error in=w1) -> ()  [unwired: 1 out]
